vi "Color Grab.vi"() -> ()   [LabVIEW 2019]
uses:
  <vilib>/userDefined/High Color/IMAQdx.ctl
  <vilib>/vision/driver/NI_Vision_Acquisition_Software.lvlib
  <vilib>/vision/NI_Vision_Development_Module.lvlib
panel:
  out "Empty":bool
  out "Yellow":bool
  out "White":bool
  out "Blue":bool
  in  "Session In":T1="cam2"
  out "Image":T2(plugin-control)
  out "Color Spectrum":dbl[](array[numeric]) format="%.2f"
  # "0"
  # "1"
  # "2"
  # "3"
  # "4"
  # "5"
  # "6"
  # "7"
  # "8"
  # "9"
  # "10"
  # "11"
  # "12"
  # "13"
  # "14"
  # "15"
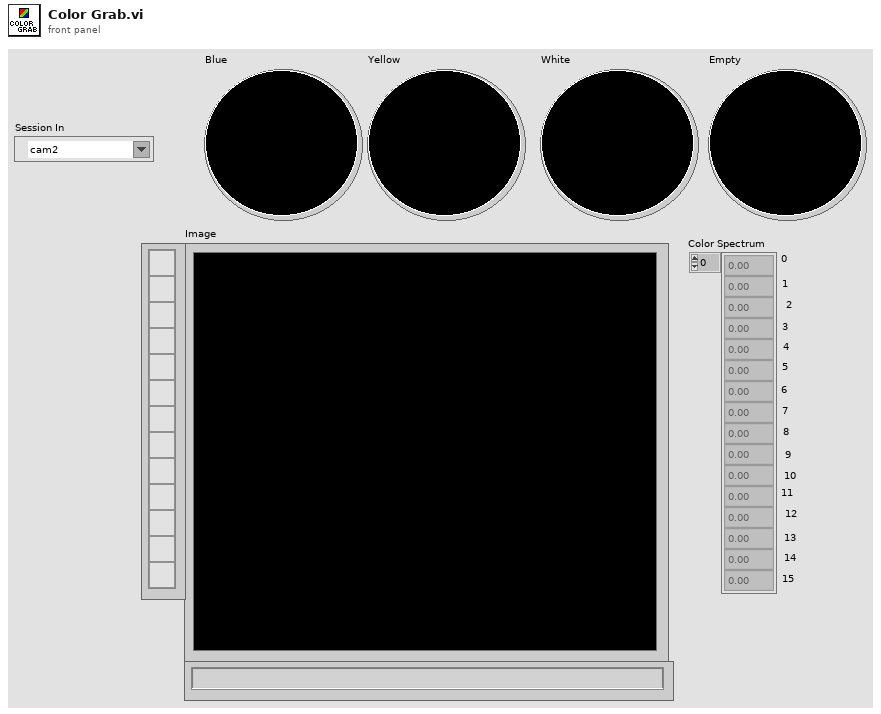
[diagram p1: front panel]
types:
  T1 = typedef "IMAQdx.ctl" = refnum<k21>
  T2 = typedef "IMAQ Image.ctl" = refnum<image>
  T3 = typedef "Image Type" = u32
  T4 = cluster{"Global Rectangle":i32[], "Contours":cluster{"Contour Type":u32, "ROI Type":u32, "Points":i32[]}[]}
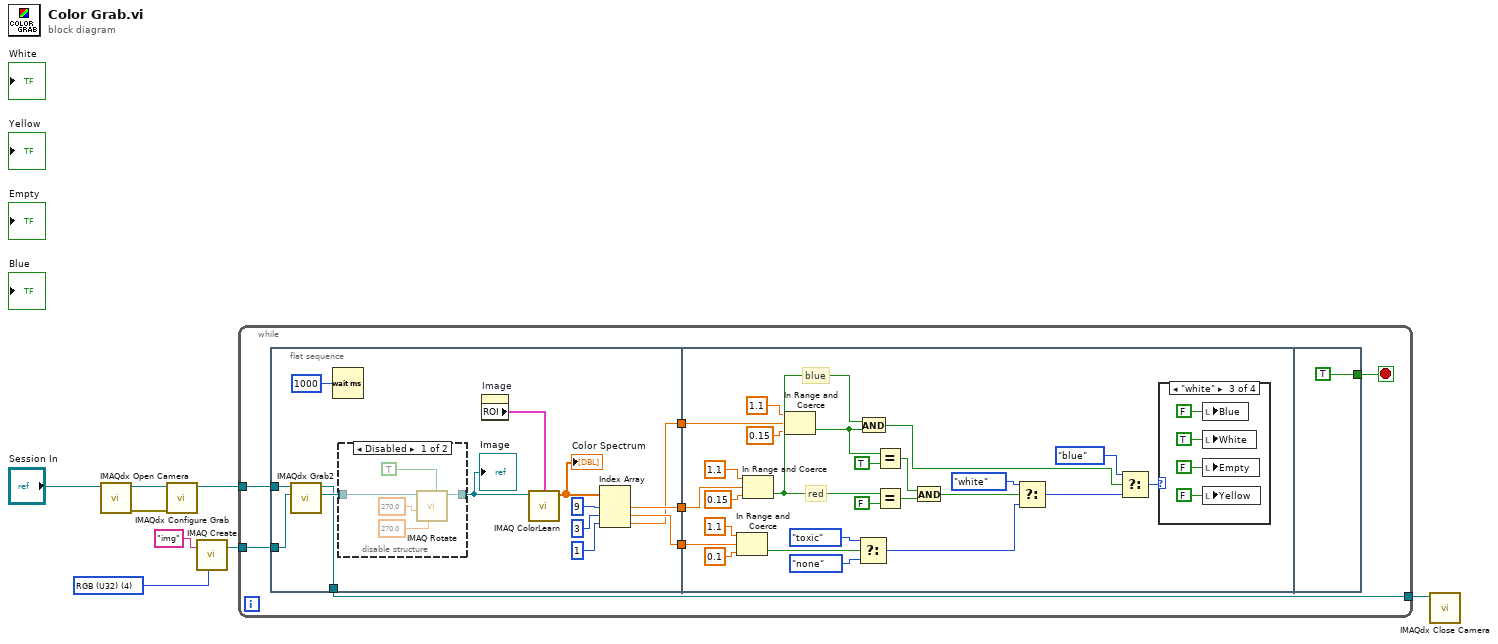
[diagram p0: block diagram]
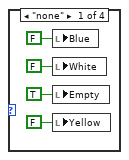
[diagram p3: hidden frame]
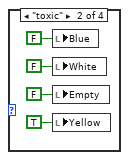
[diagram p4: hidden frame]
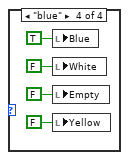
[diagram p5: hidden frame]
diagram:
  w2 = T3 4 items=["Grayscale (U8)", "Grayscale (I16)", "Grayscale (SGL)", "Complex (CSG)", "RGB (U32)", "HSL (U32)", "RGB (U64)", "Grayscale (U16)"] ("Image Type")
  n1 = call <vilib>:"IMAQdx Open Camera.vi"("Session In"="Session In") -> ("error out"=w7:errorcluster, "Session Out"=w6:T1)  [unwired: 9 in]
  n2 = call <vilib>:"IMAQdx Configure Grab.vi"("error in"=w7, "Session In"=w6) -> ("Session Out"=w5:T1)  [unwired: 8 in, 1 out]
  n3 = call "IMAQ Create"("Image Name"="img", "Image Type"=w2) -> ("New Image"=w4:T2)  [unwired: 3 in, 1 out]
  n4 = while {
    tunnel: w5 -> [w15]
    tunnel: w4 -> [w14]
    tunnel: [w13] -> w1
    stop <- w9 stop-if-true
    n5 = flat-sequence {
      tunnel: w15 -> [w29]
      tunnel: w14 -> [w28]
      tunnel: [w18] -> w13
      tunnel: [w25] -> w12
      tunnel: [w23] -> w11
      tunnel: [w21] -> w10
      tunnel: w12 -> [w42]
      tunnel: w11 -> [w45]
      tunnel: w10 -> [w48]
      tunnel: [TRUE] -> w9
      frame #0 {
        n6 = call <vilib>:"IMAQdx Grab2.vi"("Image In"=w28, "Session In"=w29) -> ("Image Out"=w27:T2, "Session Out"=w18:T1)  [unwired: 6 in, 2 out]
        n7 = Wait (ms)(milliseconds to wait=u32 1000) -> ()  [unwired: 1 out]
        n8 = disable-structure shown="Disabled" {
          disable-tunnel: w27 -> [w34 w35]
          disable-tunnel: [w33 w35] -> w19
          frame Disabled {
            n9 = call "IMAQ Rotate"("Maintain Size"=TRUE, "Replace Value"=sgl 270.0, "Angle (degrees)"=sgl 270.0, "Image Src"=w34) -> ("Image Dst Out"=w33:T2)  [unwired: 6 in, 1 out]
          }
          frame Enabled {
          }
        }
        "Image" <- w19
        n10 = property on="Image" class="ImageControl"() -> ("ROI"=w17:T4)  [unwired: 2 in, 2 out]
        n11 = call "IMAQ ColorLearn"("ROI Descriptor"=w17, "Image"=w19) -> ("Color Spectrum"=w20:dbl[])  [unwired: 6 in, 1 out]
        "Color Spectrum" <- w20
        n12 = Index Array(array=w20, index #1=9 ("index"), index #2=3 ("index"), index #3=1 ("index")) -> (element #1=w25:dbl, element #2=w23:dbl, element #3=w21:dbl)
      }
      frame #1 {
        # "blue"
        # "red"
        n13 = In Range and Coerce(upper limit=1.1, x=w45, lower limit=0.1) -> (In Range?=w39:bool)  [unwired: 1 out]
        n14 = In Range and Coerce(upper limit=1.1, x=w42, lower limit=0.15) -> (In Range?=w55:bool)  [unwired: 1 out]
        n15 = In Range and Coerce(upper limit=1.1, x=w48, lower limit=0.15) -> (In Range?=w54:bool)  [unwired: 1 out]
        n16 = Select(t=enum16{"blue", "white", "toxic", "none"}."toxic", s=w39, f=enum16{"blue", "white", "toxic", "none"}."none") -> (s? t:f=w38:enum16{"blue", "white", "toxic", "none"})
        n17 = And(x=w55, y=w54) -> (x .and. y?=w53:bool)
        n18 = Equal?(x=w54, y=TRUE) -> (x = y?=w57:bool)
        n19 = Equal?(x=w55, y=FALSE) -> (x = y?=w56:bool)
        n20 = And(x=w57, y=w56) -> (x .and. y?=w58:bool)
        n21 = Select(t=enum16{"blue", "white", "toxic", "none"}."white", s=w58, f=w38) -> (s? t:f=w59:enum16{"blue", "white", "toxic", "none"})
        n22 = Select(t=enum16{"blue", "white", "toxic", "none"}."blue", s=w53, f=w59) -> (s? t:f=w60:enum16{"blue", "white", "toxic", "none"})
        n23 = case shown="\"white\"" w60 {
          frame "none" {
            n24 = local write "Blue"(FALSE ("Blue")) -> ()
            n25 = local write "White"(FALSE ("White")) -> ()
            n26 = local write "Empty"(TRUE ("Empty")) -> ()
            n27 = local write "Yellow"(FALSE ("Yellow")) -> ()
          }
          frame "toxic" {
            n28 = local write "Blue"(FALSE ("Blue")) -> ()
            n29 = local write "White"(FALSE ("White")) -> ()
            n30 = local write "Empty"(FALSE ("Empty")) -> ()
            n31 = local write "Yellow"(TRUE ("Yellow")) -> ()
          }
          frame "white" {
            n32 = local write "Blue"(FALSE ("Blue")) -> ()
            n33 = local write "White"(TRUE ("White")) -> ()
            n34 = local write "Empty"(FALSE ("Empty")) -> ()
            n35 = local write "Yellow"(FALSE ("Yellow")) -> ()
          }
          frame "blue" {
            n36 = local write "Blue"(TRUE ("Blue")) -> ()
            n37 = local write "White"(FALSE ("White")) -> ()
            n38 = local write "Empty"(FALSE ("Empty")) -> ()
            n39 = local write "Yellow"(FALSE ("Yellow")) -> ()
          }
        }
      }
      frame #2 {
      }
    }
  }
  n40 = call <vilib>:"IMAQdx Close Camera.vi"("Session In"=w1) -> ()  [unwired: 10 in, 1 out]
